vi "increment.vi"(10 "i":i32) -> (2 "i++":i32)   [LabVIEW 2024]
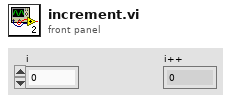
[diagram p1: front panel]
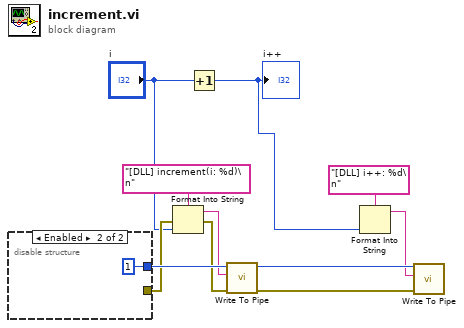
[diagram p0: block diagram]
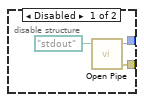
[diagram p2: hidden frame]
diagram:
  n1 = disable-structure shown="Enabled" {
    disable-tunnel: [w13 1 ("file descriptor")] -> w11
    disable-tunnel: [w12 _] -> w9
    frame Disabled {
      n2 = call <vilib>:"Open Pipe.vi"("path to named pipe"=path "stdout") -> ("error out"=w12:errorcluster, "file descriptor"=w13:i32)  [unwired: 3 in]
    }
    frame Enabled {
    }
  }
  n3 = Format Into String(format string="[DLL] increment(i: %d)\n", error in=w9, "i") -> (resulting string=w7:string, error out=w8:errorcluster)  [unwired: 1 in]
  n4 = Increment(x="i") -> (x+1=w1:i32)
  "i++" <- w1
  n5 = call <vilib>:"Write To Pipe.vi"("error in (no error)"=w8, "data"=w7, "file descriptor"=w11) -> ("error out"=w5:errorcluster, "file descriptor"=w6:i32)  [unwired: 2 in, 1 out]
  n6 = Format Into String(format string="[DLL] i++: %d\n", w1) -> (resulting string=w3:string)  [unwired: 2 in, 1 out]
  n7 = call <vilib>:"Write To Pipe.vi"("error in (no error)"=w5, "data"=w3, "file descriptor"=w6) -> ()  [unwired: 2 in, 3 out]
